vi "SoundEffects.vi"(0 "Gyro Data":T1, 1 "Numeric Control":i32) -> ()   [LabVIEW 2021]
doc: "Responsible for the generation of sound effects when corresponding events occur"
uses:
  globals/WeaponChanged_glob.vi
  globals/MotionDetected_glob.vi
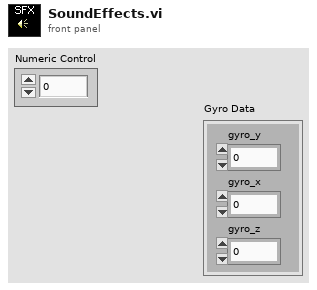
[diagram p1: front panel]
types:
  T1 = cluster{"gyro_y":dbl, "gyro_x":dbl, "gyro_z":dbl}
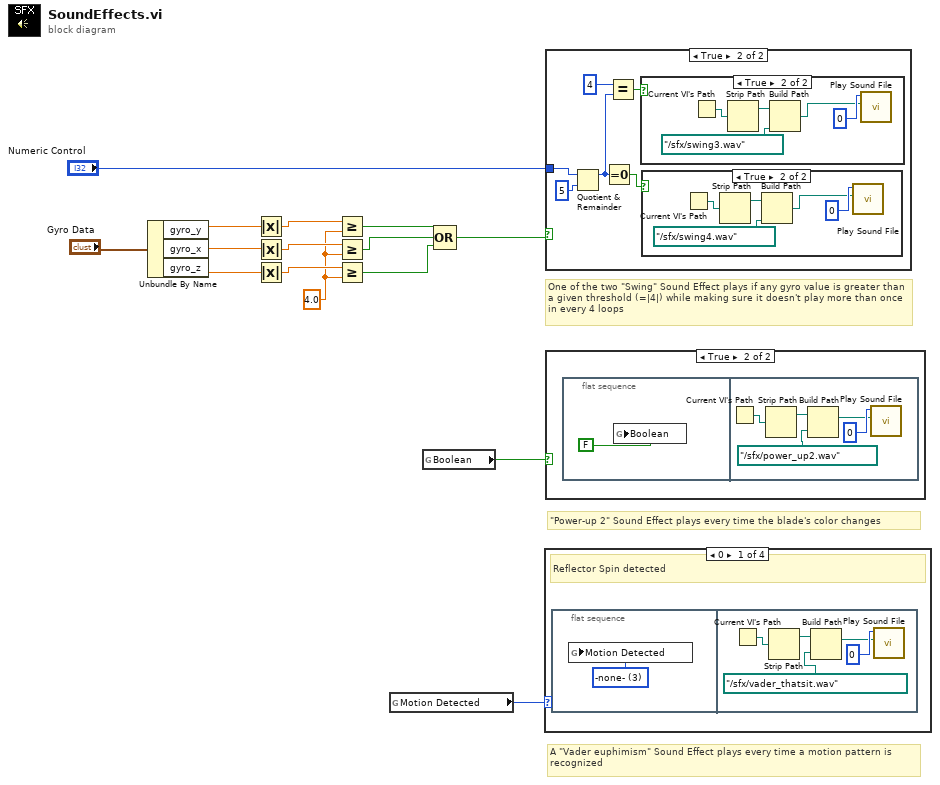
[diagram p0: block diagram]
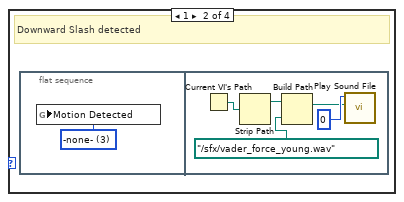
[diagram p2: hidden frame]
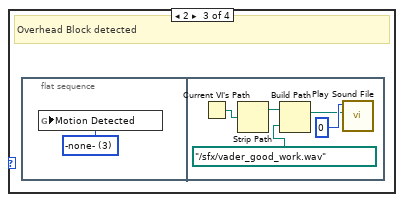
[diagram p3: hidden frame]
diagram:
  w8 = 4.0 ("y")
  # "A \"Vader euphimism\" Sound Effect plays every time a motion pattern is recognized"
  # "\"Power-up 2\" Sound Effect plays every time the blade's color changes"
  # "One of the two \"Swing\" Sound Effect plays if any gyro value is greater than a given threshold (=|4|) while making sure it doesn't play more than once in every 4 loops"
  n1 = Unbundle By Name("Gyro Data") -> ("gyro_y"=w6:dbl, "gyro_x"=w5:dbl, "gyro_z"=w4:dbl)
  n2 = Absolute Value(x=w6) -> (abs(x)=w9:dbl)
  n3 = Absolute Value(x=w5) -> (abs(x)=w10:dbl)
  n4 = Absolute Value(x=w4) -> (abs(x)=w11:dbl)
  n5 = Greater Or Equal?(x=w9, y=w8) -> (x >= y?=w12:bool)
  n6 = Greater Or Equal?(x=w10, y=w8) -> (x >= y?=w13:bool)
  n7 = Greater Or Equal?(x=w11, y=w8) -> (x >= y?=w14:bool)
  n8 = global read "MotionDetected_glob.vi" "Motion Detected"() -> (w1:u16)
  n9 = global read "WeaponChanged_glob.vi" "Boolean"() -> (w15:bool)
  n10 = Compound Arithmetic op=OR(w12, w13, w14) -> (w3:bool)
  n11 = case shown="0" w1 {
    frame 0 {
      # "Reflector Spin detected"
      n12 = flat-sequence {
        frame #0 {
          w16 = u16 3 items=["reflector spin", "downward slash", "overhead block", "-none-"] ("Motion Detected")
          n13 = global write "MotionDetected_glob.vi" "Motion Detected"(w16) -> ()
        }
        frame #1 {
          n14 = Current VI's Path() -> (path=w21:path)
          n15 = Strip Path(path=w21) -> (stripped path=w20:path)  [unwired: 1 out]
          n16 = Build Path(base path=w20, name or relative path=path "../sfx/vader_thatsit.wav" ("path")) -> (appended path=w18:path)
          n17 = call <vilib>:"Play Sound File.vi"("path"=w18, "device ID"=u32 0) -> ()  [unwired: 8 in, 2 out]
        }
      }
    }
    frame 1 {
      # "Downward Slash detected"
      n18 = flat-sequence {
        frame #0 {
          w22 = u16 3 items=["reflector spin", "downward slash", "overhead block", "-none-"] ("Motion Detected")
          n19 = global write "MotionDetected_glob.vi" "Motion Detected"(w22) -> ()
        }
        frame #1 {
          n20 = Current VI's Path() -> (path=w27:path)
          n21 = Strip Path(path=w27) -> (stripped path=w26:path)  [unwired: 1 out]
          n22 = Build Path(base path=w26, name or relative path=path "../sfx/vader_force_young.wav" ("path")) -> (appended path=w24:path)
          n23 = call <vilib>:"Play Sound File.vi"("path"=w24, "device ID"=u32 0) -> ()  [unwired: 8 in, 2 out]
        }
      }
    }
    frame 2 {
      # "Overhead Block detected"
      n24 = flat-sequence {
        frame #0 {
          w28 = u16 3 items=["reflector spin", "downward slash", "overhead block", "-none-"] ("Motion Detected")
          n25 = global write "MotionDetected_glob.vi" "Motion Detected"(w28) -> ()
        }
        frame #1 {
          n26 = Current VI's Path() -> (path=w33:path)
          n27 = Strip Path(path=w33) -> (stripped path=w32:path)  [unwired: 1 out]
          n28 = Build Path(base path=w32, name or relative path=path "../sfx/vader_good_work.wav" ("path")) -> (appended path=w30:path)
          n29 = call <vilib>:"Play Sound File.vi"("path"=w30, "device ID"=u32 0) -> ()  [unwired: 8 in, 2 out]
        }
      }
    }
    frame 3, Default {
    }
  }
  n30 = case shown="True" w3 {
    tunnel: "Numeric Control" -> [_ w39]
    frame False {
    }
    frame True {
      n31 = Quotient & Remainder(x=w39, y=5) -> (x-y*floor(x/y)=w36:i32)  [unwired: 1 out]
      n32 = Equal To 0?(x=w36) -> (x = 0?=w38:bool)
      n33 = Equal?(x=4, y=w36) -> (x = y?=w35:bool)
      n34 = case shown="True" w35 {
        frame False {
        }
        frame True {
          n35 = Current VI's Path() -> (path=w44:path)
          n36 = Strip Path(path=w44) -> (stripped path=w43:path)  [unwired: 1 out]
          n37 = Build Path(base path=w43, name or relative path=path "../sfx/swing3.wav" ("path")) -> (appended path=w41:path)
          n38 = call <vilib>:"Play Sound File.vi"("path"=w41, "device ID"=u32 0) -> ()  [unwired: 8 in, 2 out]
        }
      }
      n39 = case shown="True" w38 {
        frame False {
        }
        frame True {
          n40 = Current VI's Path() -> (path=w49:path)
          n41 = Strip Path(path=w49) -> (stripped path=w48:path)  [unwired: 1 out]
          n42 = Build Path(base path=w48, name or relative path=path "../sfx/swing4.wav" ("path")) -> (appended path=w46:path)
          n43 = call <vilib>:"Play Sound File.vi"("path"=w46, "device ID"=u32 0) -> ()  [unwired: 8 in, 2 out]
        }
      }
    }
  }
  n44 = case shown="True" w15 {
    frame False {
    }
    frame True {
      n45 = flat-sequence {
        frame #0 {
          n46 = global write "WeaponChanged_glob.vi" "Boolean"(FALSE ("Boolean")) -> ()
        }
        frame #1 {
          n47 = Current VI's Path() -> (path=w55:path)
          n48 = Strip Path(path=w55) -> (stripped path=w54:path)  [unwired: 1 out]
          n49 = Build Path(base path=w54, name or relative path=path "../sfx/power_up2.wav" ("path")) -> (appended path=w52:path)
          n50 = call <vilib>:"Play Sound File.vi"("path"=w52, "device ID"=u32 0) -> ()  [unwired: 8 in, 2 out]
        }
      }
    }
  }
